vi "계산기2.vi"() -> ()   [LabVIEW 2018]
panel:
  out "문자열":string
  in  "취소 버튼":bool
  in  "=":bool
  in  ".":bool
  in  "0":bool
  in  "+/-":bool
  in  "+":bool
  in  "3":bool
  in  "2":bool
  in  "1":bool
  in  "-":bool
  in  "6":bool
  in  "5":bool
  in  "4":bool
  in  "X":bool
  in  "9":bool
  in  "8":bool
  in  "7":bool
  in  "/":bool
  in  "x^(1/2)":bool
  in  "x^2":bool
  in  "1/x":bool
  in  "CLR":bool
  in  "C":bool
  in  "CE":bool
  in  "%":bool
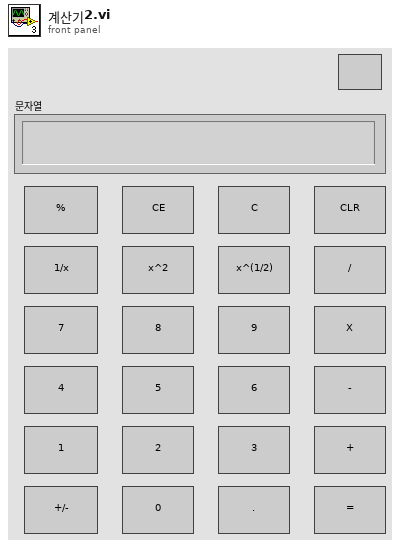
[diagram p1: front panel]
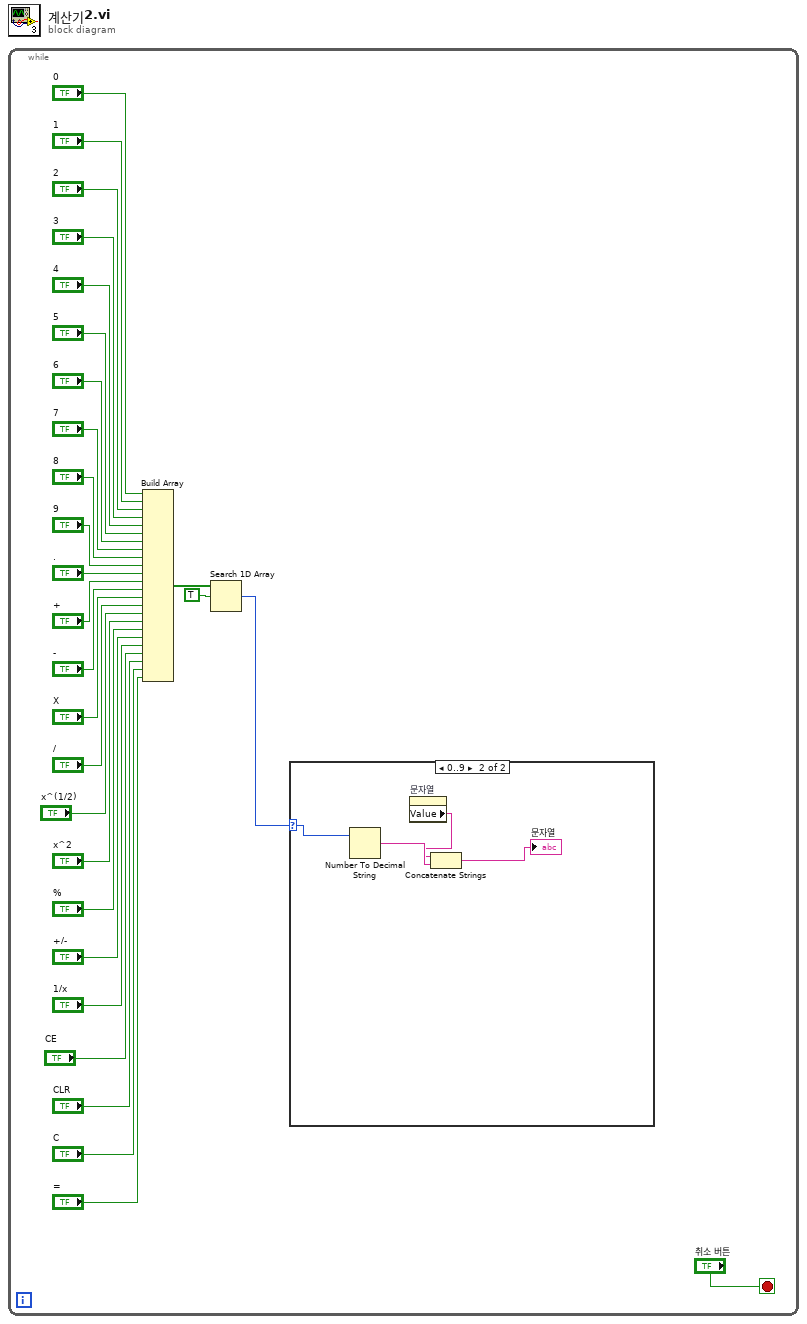
[diagram p0: block diagram]
diagram:
  n1 = while {
    stop <- "취소 버튼" stop-if-true
    n2 = Build Array("0", "1", "2", "3", "4", "5", "6", "7", "8", "9", ".", "+", "-", "X", "/", "x^(1/2)", "x^2", "%", "+/-", "1/x", "CE", "CLR", "C", "=") -> (w28:bool[])
    n3 = Search 1D Array(1D array=w28, element=TRUE) -> (index of element=w2:i32)  [unwired: 1 in]
    n4 = case shown="0..9" w2 {
      selector: w2 -> [_ w32]
      frame 0, Default {
      }
      frame 0..9 {
        n5 = Number To Decimal String(number=w32) -> (decimal integer string=w31:string)  [unwired: 1 in]
        n6 = property on="문자열" class="Str"() -> ("Value"=w29:string)  [unwired: 2 in, 2 out]
        n7 = Concatenate Strings(w29, w31) -> (→"문자열":string)
      }
    }
  }
